vi "Actor Core.vi"(8 "error in":errorcluster, 11 "Thermocouples in":refnum<class "Thermocouples.lvclass">) -> (0 "error out":errorcluster, 3 "Actor out":refnum<class "Actor.lvclass">)   [LabVIEW 2015, in "AMS UI.lvlib" / "Thermocouples.lvclass"]
doc: "(<B>Filename</B>: Actor Framework.lvlib:Actor.lvclass:Actor Core.vi)\n\nReceives messages to the actor, reacts to them, and initiates any error handling that may shut the actor down.\n\nDescendant classes may override this VI to append parallel tasks for the actor to complete while it handles messages. Overrides use the Call Parent Method node."
uses:
  Thermocouples.lvclass
  <vilib>/ActorFramework/Actor/Actor.lvclass
  <vilib>/ActorFramework/Actor/Actor.lvclass/Actor.ctl
  <vilib>/ActorFramework/Message Enqueuer/Message Enqueuer.lvclass/Message Enqueuer.ctl
  Thermocouples.lvclass/Thermocouples.ctl
  <vilib>/ActorFramework/Message Enqueuer/Init from Existing Queue.vi
  <vilib>/ActorFramework/Message Enqueuer/Message Enqueuer.lvclass
  AMS Gas Actor/AMS Gas Actor.lvclass
  eActor/eActor.lvclass
panel:
  out "Waveform Chart":T1(graph)
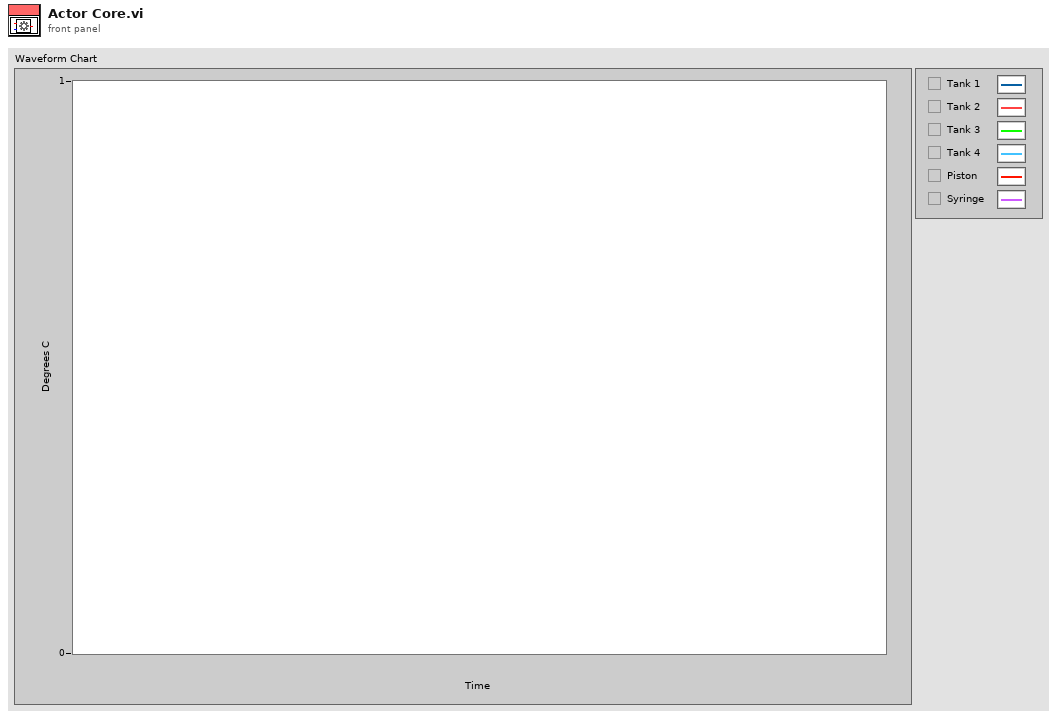
[diagram p1: front panel]
types:
  T1 = cluster{"Double":dbl, "Double":dbl, "Double":dbl, "Double":dbl, "Double":dbl, "Double":dbl}
  T2 = enum32{"Invalid", "Standard", "Closed", "Hidden", "Minimized", "Maximized"}
  T3 = cluster{"Double":dbl, "Double":dbl, "Double":dbl, "Double":dbl, "Double":dbl, "Double":dbl}[]
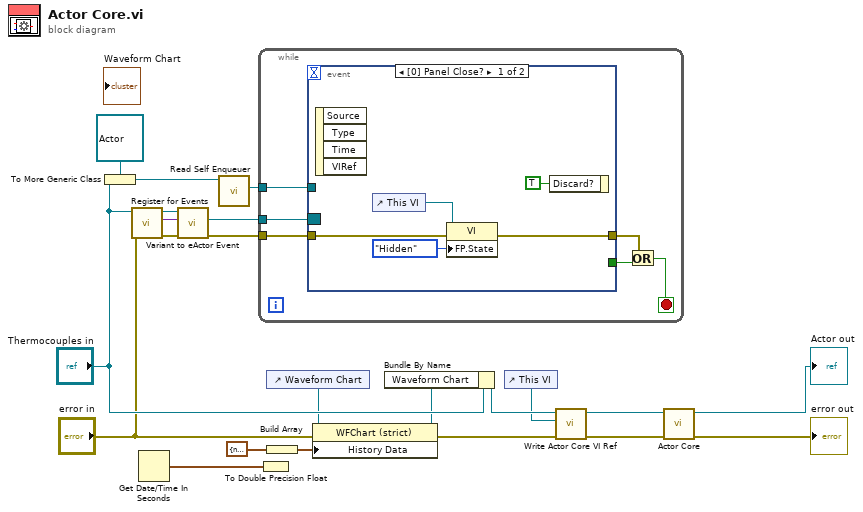
[diagram p0: block diagram]
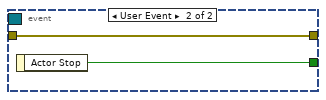
[diagram p2: hidden frame]
diagram:
  n1 = To More Generic Class(target class=refnum<class "Actor.lvclass"> refnum ("Actor"), reference="Thermocouples in") -> (generic class reference=w18:refnum<class "Actor.lvclass">)
  n2 = call-dynamic "Register for Events.vi"("error in (no error)"="error in", "eActor in"="Thermocouples in") -> ("error out"=w8:errorcluster, "Event Registration Refnum"=w20:variant, "eActor out"=w6:refnum<class "Thermocouples.lvclass">)  [unwired: 7 in]
  n3 = Get Date/Time In Seconds() -> (seconds since 1Jan1904=w12:timestamp)
  n4 = call "Variant to eActor Event.vi"("error in (no error)"=w8, "Variant"=w20, "eActor in"=w6) -> ("error out"=w7:errorcluster, "Event Registration Refnum"=w9:refnum<event-registration>)  [unwired: 6 in, 1 out]
  n5 = call <vilib>:"Read Self Enqueuer.vi"("Actor"=w18) -> ("Self Enqueuer"=w19:refnum<class "Message Enqueuer.lvclass">)  [unwired: 10 in]
  n6 = while {
    tunnel: w7 -> [w27]
    tunnel: w9 -> [w28]
    tunnel: w19 -> [w25]
    stop <- w23 stop-if-true
    n7 = event shown="[0] Panel Close?" {
      selector: w28 -> [_ _]
      dyn-events: _ -> [_ _]
      timeout: _ -> [_ _]
      tunnel: w27 -> [w32 w34]
      tunnel: [_ w35] -> w26
      tunnel: w25 -> [_ _]
      tunnel: [w29 w34] -> w24
      event Panel Close? {
        n8 = event-data() -> ()  [unwired: 1 in, 4 out]
        n9 = control-ref of="This VI"() -> (w31:refnum<vi>)
        n10 = property class="VI"(reference=w31, error in=w32, "FP.State"=T2."Hidden" ("Front Panel Window:State")) -> (error out=w29:errorcluster)  [unwired: 1 out]
        n11 = event-data("Discard?"=TRUE) -> ()  [unwired: 1 in, 1 out]
      }
      event User Event {
        n12 = event-data() -> ("Actor Stop"=w35:bool)  [unwired: 1 in]
      }
    }
    n13 = Or(x=w24, y=w26) -> (x .or. y?=w23:bool)
  }
  n14 = To Double Precision Float(number=w12) -> ()  [unwired: 1 out]
  n15 = control-ref of="Waveform Chart"() -> (w11:refnum<vi>)
  n16 = Build Array(T1 {"Double"=nan, "Double"=nan, "Double"=nan, "Double"=nan, "Double"=nan, "Double"=nan} ("output cluster")) -> (w13:T3)
  n17 = property class="WFChart (strict)"(reference=w11, error in="error in", "History Data"=w13) -> (reference out=w10:refnum<vi>, error out=w3:errorcluster)
  n18 = Bundle By Name(cluster="Thermocouples in", "Waveform Chart"=w10) -> (w5:refnum<class "Thermocouples.lvclass">)
  n19 = control-ref of="This VI"() -> (w1:refnum<vi>)
  n20 = call "Write Actor Core VI Ref.vi"("error in (no error)"=w3, "Actor Core VI Ref"=w1, "AMS Gas Actor in"=w5) -> ("error out"=w2:errorcluster, "AMS Gas Actor out"=w4:refnum<class "Thermocouples.lvclass">)  [unwired: 7 in]
  n21 = call-parent "Actor Core.vi"("error in"=w2, "Actor in"=w4) -> ("error out"=→"error out":errorcluster, "Actor out"=→"Actor out":refnum<class "Actor.lvclass">)  [unwired: 8 in]
